vi "P841CW.vi"(4 "Special Function In":string, 6 "Velocity":dbl, 7 "Abort":refnum<vi>, 8 "Axis":bool[](array[boolean]), 9 "Positions":dbl[](array[numeric]), 10 "Action":T1=enum."MVR", 11 "VISA In":refnum<visa-resource-name>) -> (0 "Special Function":string, 1 "Status":bool, 2 "Position Out":dbl[](array[numeric]), 3 "VISA Out":refnum<visa-resource-name>)   [LabVIEW 2014]
uses:
  Controls/StageStates.ctl
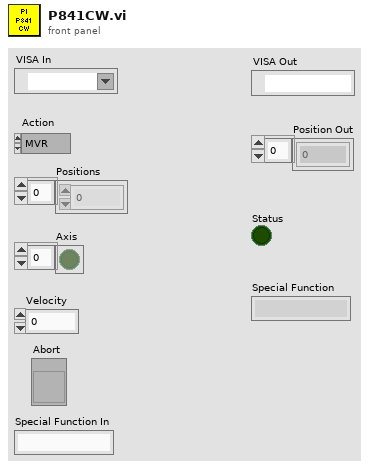
[diagram p1: front panel]
types:
  T1 = typedef "StageStates.ctl" = enum16{"POSITION", "MVR", "MOVE", "HALT", "ONTARGET", "ERROR", "EXIT", "HOME", "ZEROPOS", "NANOPOS", "QUIT", "ANALOG"}
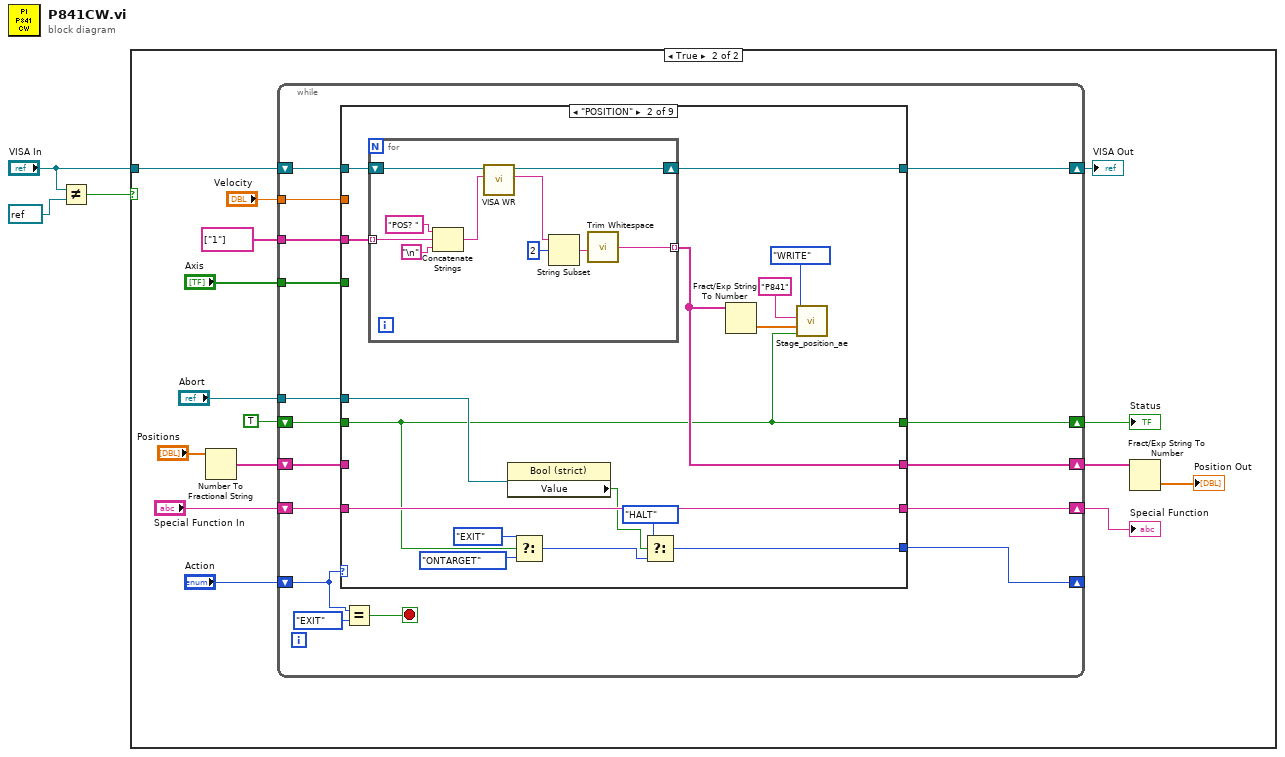
[diagram p0: block diagram]
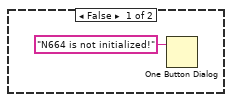
[diagram p2: hidden frame]
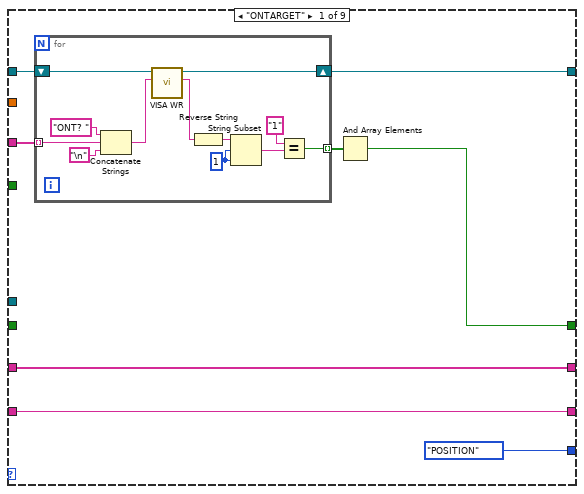
[diagram p3: hidden frame]
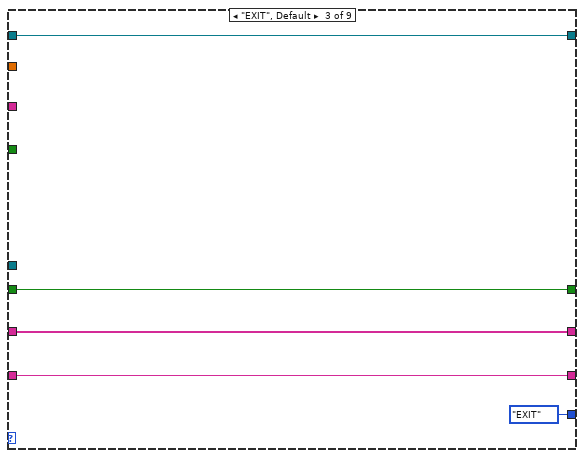
[diagram p4: hidden frame]
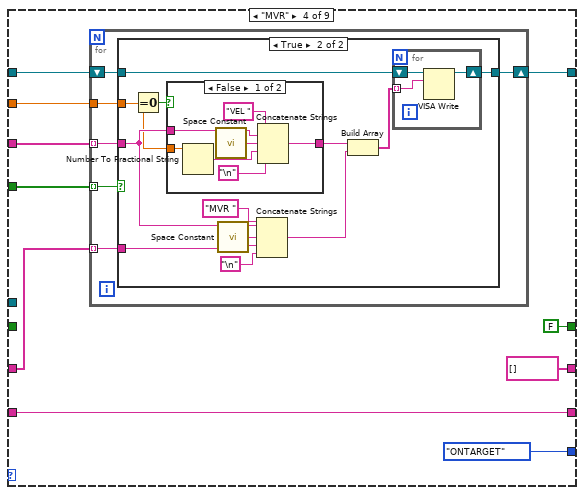
[diagram p5: hidden frame]
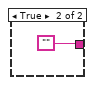
[diagram p7: hidden frame]
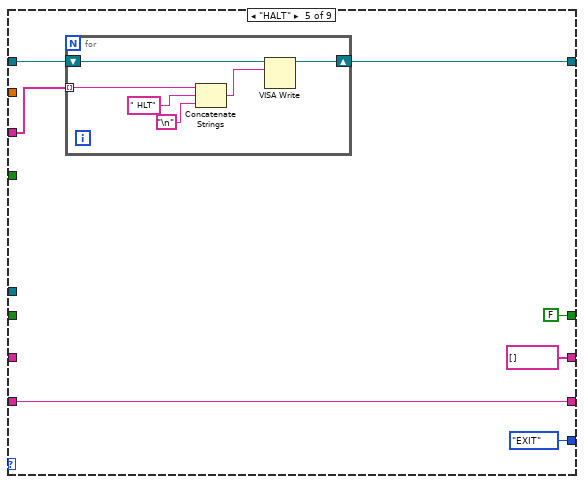
[diagram p8: hidden frame]
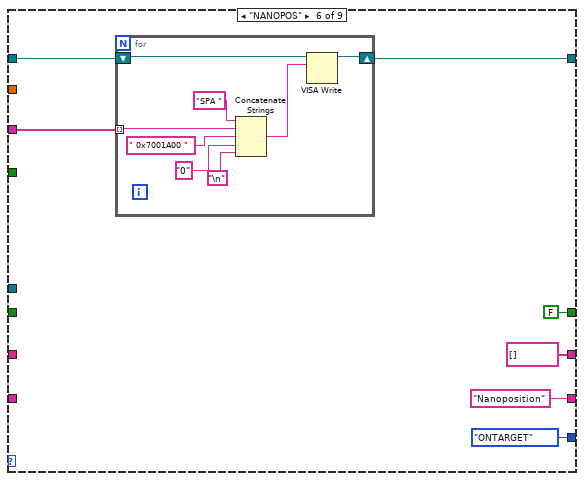
[diagram p9: hidden frame]
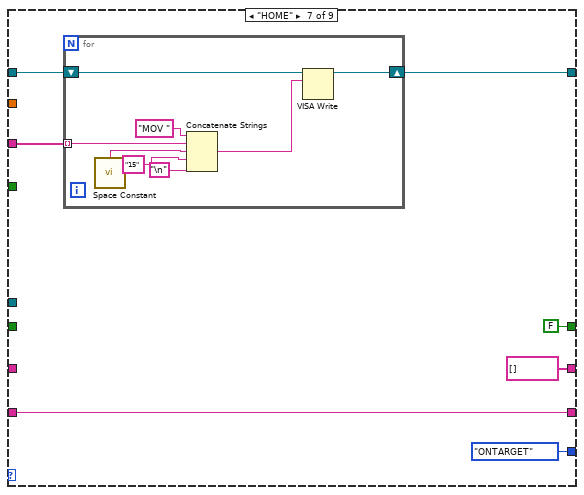
[diagram p10: hidden frame]
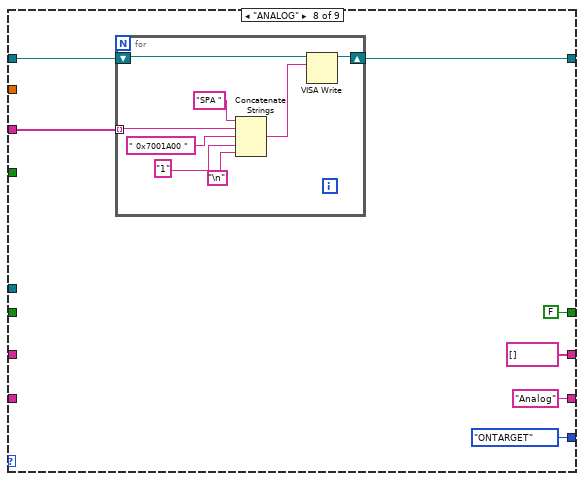
[diagram p11: hidden frame]
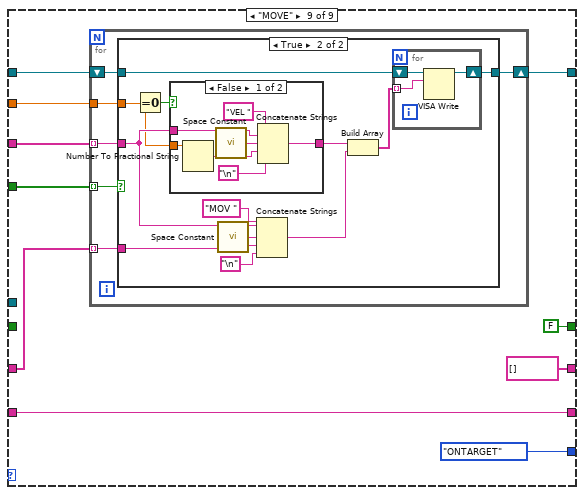
[diagram p12: hidden frame]
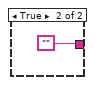
[diagram p14: hidden frame]
diagram:
  n1 = Not Equal?(x="VISA In", y=refnum<visa-resource-name> refnum ("VISA In")) -> (x != y?=w1:bool)
  n2 = case shown="True" w1 {
    tunnel: "VISA In" -> [_ w19]
    frame False {
      n3 = One Button Dialog(message="N664 is not initialized!") -> ()  [unwired: 1 in, 1 out]
    }
    frame True {
      n4 = Number To Fractional String(number="Positions") -> (F-format string=w13:string[])  [unwired: 3 in]
      n5 = while {
        tunnel: string[] ["1"] -> [w35]
        shift-right: [w25] -> _
        shift-left: "Action" -> [w29]
        shift-right: [w32] -> w12
        shift-left: w13 -> [w33]
        shift-right: [w30] -> w17
        shift-left: TRUE -> [w31]
        tunnel: "Axis" -> [w28]
        tunnel: "Velocity" -> [w26]
        shift-right: [w23] -> w9
        shift-left: "Special Function In" -> [w24]
        shift-right: [w21] -> w6
        shift-left: w19 -> [w34]
        tunnel: "Abort" -> [w20]
        stop <- w22 stop-if-true
        n6 = case shown="\"POSITION\"" w29 {
          tunnel: w35 -> [w42 w70 _ w95 w133 w145 w161 w175 w193]
          tunnel: w34 -> [w43 w71 w86 w96 w132 w146 w160 w176 w194]
          tunnel: w33 -> [w40 _ w84 w94 _ _ _ _ w192]
          tunnel: [w40 w60 w84 string[] [] string[] [] string[] [] string[] [] string[] [] string[] []] -> w32
          tunnel: w31 -> [_ w56 w85 _ _ _ _ _ _]
          tunnel: [w38 w56 w85 FALSE FALSE FALSE FALSE FALSE FALSE] -> w30
          tunnel: w28 -> [_ _ _ w93 _ _ _ _ w191]
          tunnel: w26 -> [_ _ _ w92 _ _ _ _ w190]
          tunnel: [StageStates."POSITION" ("Action") w59 StageStates."EXIT" ("Action") StageStates."ONTARGET" ("Action") StageStates."EXIT" ("Action") StageStates."ONTARGET" ("Action") StageStates."ONTARGET" ("Action") StageStates."ONTARGET" ("Action") StageStates."ONTARGET" ("Action")] -> w25
          tunnel: w24 -> [w39 w69 w83 w90 w131 _ w159 _ w189]
          tunnel: [w39 w69 w83 w90 w131 "Nanoposition" w159 "Analog" w189] -> w23
          tunnel: [w37 w68 w86 w89 w129 w142 w155 w170 w188] -> w21
          tunnel: w20 -> [_ w57 _ _ _ _ _ _ _]
          frame "ONTARGET" {
            n7 = for {
              tunnel: w42 -> [w54] mode=indexing
              tunnel: [w50] -> w41 mode=indexing
              shift-right: [w44] -> w37
              shift-left: w43 -> [w55]
              w46 = 1 ("length (rest)")
              n8 = Concatenate Strings("ONT? " ("string"), w54, "\n") -> (w45:string)
              n9 = call "VISA WR.vi"("write buffer"=w45, "VISA Refnum in"=w55) -> ("read buffer"=w53:string, "VISA Refnum out"=w44:refnum<visa-resource-name>)  [unwired: 7 in, 1 out]
              n10 = Reverse String(1:w53) -> (0:w47:string)
              n11 = String Subset(string=w47, offset (0)=w46, length (rest)=w46) -> (substring=w52:string)
              n12 = Equal?(x="1", y=w52) -> (x = y?=w50:bool)
            }
            n13 = And Array Elements(Boolean array=w41) -> (logical AND=w38:bool)
          }
          frame "POSITION" {
            n14 = for {
              tunnel: w70 -> [w80] mode=indexing
              tunnel: [w78] -> w60 mode=indexing
              shift-right: [w72] -> w68
              shift-left: w71 -> [w81]
              n15 = Concatenate Strings("POS? " ("string"), w80, "\n") -> (w73:string)
              n16 = call "VISA WR.vi"("write buffer"=w73, "VISA Refnum in"=w81) -> ("read buffer"=w79:string, "VISA Refnum out"=w72:refnum<visa-resource-name>)  [unwired: 7 in, 1 out]
              n17 = String Subset(string=w79, offset (0)=2) -> (substring=w74:string)  [unwired: 1 in]
              n18 = call <vilib>:"Trim Whitespace.vi"("string"=w74) -> ("trimmed string"=w78:string)  [unwired: 1 in]
            }
            n19 = property class="Bool (strict)"(reference=w57) -> ("Value"=w58:bool)  [unwired: 1 in, 2 out]
            n20 = Select(t=StageStates."EXIT" ("Action"), s=w56, f=StageStates."ONTARGET" ("Action")) -> (s? t:f=w66:T1)
            n21 = Select(t=StageStates."HALT", s=w58, f=w66) -> (s? t:f=w59:T1)
            n22 = Fract/Exp String To Number(string=w60) -> (number=w61:dbl[])  [unwired: 3 in, 1 out]
            n23 = call "Stage_position_ae.vi"("Status In"=w56, "Position In"=w61, "StageID"="P841", "Enum"=enum16{"WRITE", "READ"}."WRITE") -> ()  [unwired: 6 in, 2 out]
          }
          frame "EXIT", Default {
          }
          frame "MVR" {
            n24 = for {
              tunnel: w95 -> [w102] mode=indexing
              tunnel: w94 -> [w101] mode=indexing
              shift-right: [w99] -> w89
              shift-left: w96 -> [w100]
              tunnel: w93 -> [w98] mode=indexing
              tunnel: w92 -> [w97]
              n25 = case shown="True" w98 {
                tunnel: w102 -> [_ w109]
                tunnel: w101 -> [_ w112]
                tunnel: w100 -> [w103 w111]
                tunnel: [w103 w110] -> w99
                tunnel: w97 -> [_ w108]
                frame False {
                }
                frame True {
                  n26 = Equal To 0?(x=w108) -> (x = 0?=w107:bool)
                  n27 = case shown="False" w107 {
                    tunnel: w109 -> [w122 _]
                    tunnel: w108 -> [w119 _]
                    tunnel: [w121 ""] -> w106
                    frame False {
                      n28 = Number To Fractional String(number=w119) -> (F-format string=w120:string)  [unwired: 3 in]
                      n29 = call <vilib>:"Space Constant.vi"() -> ("String"=w125:string)
                      n30 = Concatenate Strings("VEL ", w122, w125, w120, "\n") -> (w121:string)
                    }
                    frame True {
                    }
                  }
                  n31 = call <vilib>:"Space Constant.vi"() -> ("String"=w113:string)
                  n32 = Concatenate Strings("MVR ", w109, w113, w112, "\n") -> (w105:string)
                  n33 = Build Array(w106, w105) -> (w104:string[])
                  n34 = for {
                    shift-right: [w117] -> w110
                    shift-left: w111 -> [w118]
                    tunnel: w104 -> [w116] mode=indexing
                    n35 = VISA Write(VISA resource name=w118, write buffer=w116) -> (VISA resource name out=w117:refnum<visa-resource-name>)  [unwired: 1 in, 2 out]
                  }
                }
              }
            }
          }
          frame "HALT" {
            n36 = for {
              tunnel: w133 -> [w136] mode=indexing
              shift-right: [w134] -> w129
              shift-left: w132 -> [w135]
              n37 = Concatenate Strings(w136, " HLT" ("string"), "\n") -> (w137:string)
              n38 = VISA Write(VISA resource name=w135, write buffer=w137) -> (VISA resource name out=w134:refnum<visa-resource-name>)  [unwired: 1 in, 2 out]
            }
          }
          frame "NANOPOS" {
            n39 = for {
              shift-right: [w150] -> w142
              shift-left: w146 -> [w151]
              tunnel: w145 -> [w149] mode=indexing
              n40 = Concatenate Strings("SPA " ("string"), w149, " 0x7001A00 " ("string"), "0", "\n") -> (w147:string)
              n41 = VISA Write(VISA resource name=w151, write buffer=w147) -> (VISA resource name out=w150:refnum<visa-resource-name>)  [unwired: 1 in, 2 out]
            }
          }
          frame "HOME" {
            n42 = for {
              tunnel: w161 -> [w165] mode=indexing
              shift-right: [w163] -> w155
              shift-left: w160 -> [w164]
              n43 = call <vilib>:"Space Constant.vi"() -> ("String"=w166:string)
              n44 = Concatenate Strings("MOV " ("string"), w165, w166, "15" ("string"), "\n") -> (w162:string)
              n45 = VISA Write(VISA resource name=w164, write buffer=w162) -> (VISA resource name out=w163:refnum<visa-resource-name>)  [unwired: 1 in, 2 out]
            }
          }
          frame "ANALOG" {
            n46 = for {
              shift-right: [w180] -> w170
              shift-left: w176 -> [w181]
              tunnel: w175 -> [w179] mode=indexing
              n47 = Concatenate Strings("SPA " ("string"), w179, " 0x7001A00 " ("string"), "1", "\n") -> (w178:string)
              n48 = VISA Write(VISA resource name=w181, write buffer=w178) -> (VISA resource name out=w180:refnum<visa-resource-name>)  [unwired: 1 in, 2 out]
            }
          }
          frame "MOVE" {
            n49 = for {
              tunnel: w193 -> [w200] mode=indexing
              tunnel: w192 -> [w199] mode=indexing
              shift-right: [w197] -> w188
              shift-left: w194 -> [w198]
              tunnel: w191 -> [w196] mode=indexing
              tunnel: w190 -> [w195]
              n50 = case shown="True" w196 {
                tunnel: w200 -> [_ w207]
                tunnel: w199 -> [_ w210]
                tunnel: w198 -> [w201 w209]
                tunnel: [w201 w208] -> w197
                tunnel: w195 -> [_ w206]
                frame False {
                }
                frame True {
                  n51 = Equal To 0?(x=w206) -> (x = 0?=w205:bool)
                  n52 = case shown="False" w205 {
                    tunnel: w207 -> [w220 _]
                    tunnel: w206 -> [w217 _]
                    tunnel: [w219 ""] -> w204
                    frame False {
                      n53 = Number To Fractional String(number=w217) -> (F-format string=w218:string)  [unwired: 3 in]
                      n54 = call <vilib>:"Space Constant.vi"() -> ("String"=w223:string)
                      n55 = Concatenate Strings("VEL ", w220, w223, w218, "\n") -> (w219:string)
                    }
                    frame True {
                    }
                  }
                  n56 = call <vilib>:"Space Constant.vi"() -> ("String"=w211:string)
                  n57 = Concatenate Strings("MOV ", w207, w211, w210, "\n") -> (w203:string)
                  n58 = Build Array(w204, w203) -> (w202:string[])
                  n59 = for {
                    shift-right: [w215] -> w208
                    shift-left: w209 -> [w216]
                    tunnel: w202 -> [w214] mode=indexing
                    n60 = VISA Write(VISA resource name=w216, write buffer=w214) -> (VISA resource name out=w215:refnum<visa-resource-name>)  [unwired: 1 in, 2 out]
                  }
                }
              }
            }
          }
        }
        n61 = Equal?(x=w29, y=StageStates."EXIT") -> (x = y?=w22:bool)
      }
      "Status" <- w17
      "Special Function" <- w9
      "VISA Out" <- w6
      n62 = Fract/Exp String To Number(string=w12) -> (number=→"Position Out":dbl[])  [unwired: 3 in, 1 out]
    }
  }
